vi "Pump Load Ctrl.vi"(8 "error in":errorcluster, 11 "Water Tunnel Results in":refnum<class "Water Tunnel Results.lvclass">) -> (0 "error out":errorcluster, 1 "Pump Load":dbl, 2 "Pump Inv U":dbl, 3 "Water Tunnel Results out":refnum<class "Water Tunnel Results.lvclass">)   [LabVIEW 2019, in "Results.lvlib" / "Water Tunnel Results.lvclass"]
uses:
  Water Tunnel Results.lvclass
  <vilib>/ErrorRing/Error Ring.xnode
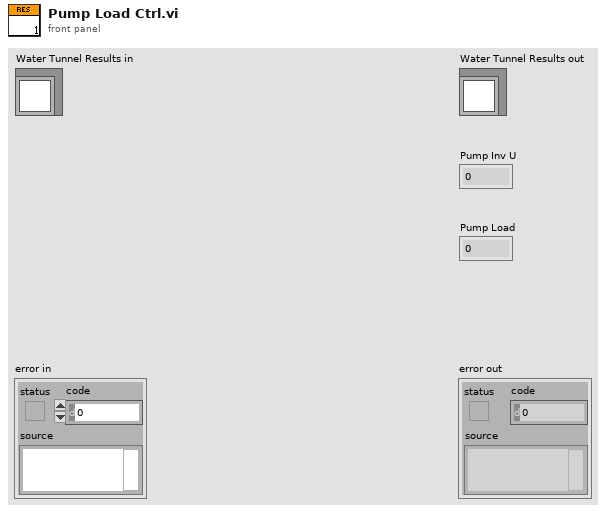
[diagram p1: front panel]
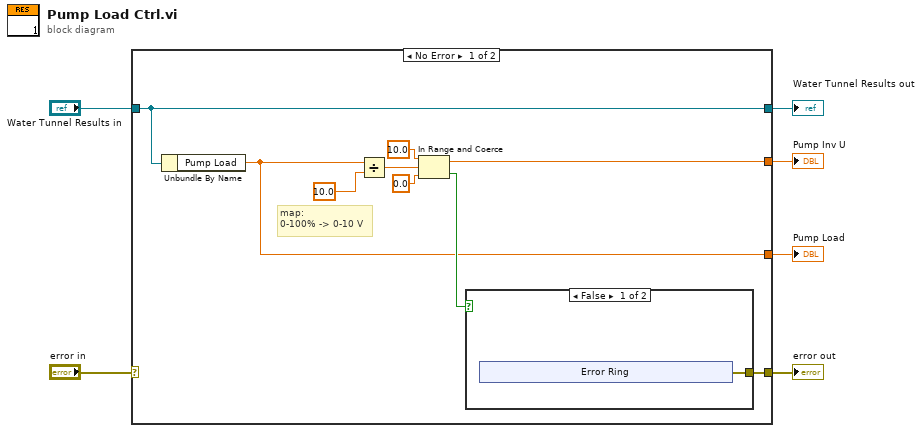
[diagram p0: block diagram]
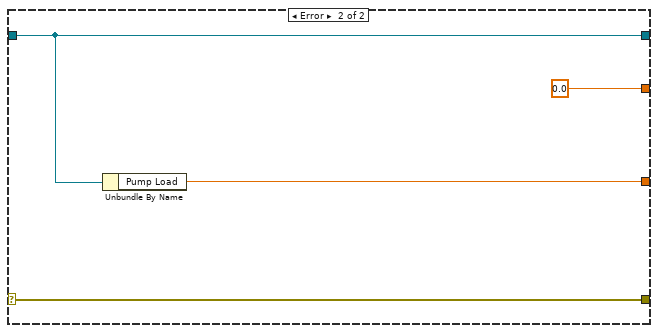
[diagram p3: hidden frame]
diagram:
  n1 = case shown="No Error" "error in" {
    selector: "error in" -> [_ w21]
    tunnel: [w8 w21] -> w5
    tunnel: [w15 w19] -> w3
    tunnel: "Water Tunnel Results in" -> [w15 w19]
    tunnel: [w10 0.0 ("upper limit")] -> w2
    tunnel: [w7 w18] -> w1
    frame No Error {
      # "map:\n0-100% -> 0-10 V"
      n2 = Unbundle By Name(w15) -> ("Pump Load"=w7:dbl)
      n3 = Divide(x=w7, y=10.0) -> (x/y=w13:dbl)
      n4 = In Range and Coerce(upper limit=10.0, x=w13, lower limit=0.0) -> (coerced(x)=w10:dbl, In Range?=w9:bool)
      n5 = case shown="False" w9 {
        tunnel: [w16 _] -> w8
        frame False {
          n6 = xnode "Error Ring"() -> ("error out"=w16:errorcluster)
        }
        frame True {
        }
      }
    }
    frame Error {
      n7 = Unbundle By Name(w19) -> ("Pump Load"=w18:dbl)
    }
  }
  "error out" <- w5
  "Water Tunnel Results out" <- w3
  "Pump Inv U" <- w2
  "Pump Load" <- w1
